vi "ep_Compute Third Current (SGL WFM).vi"(0 "current waveforms in":waveform(sgl)[](array[waveform]), 5 "wiring":T1, 11 "error in (no error)":errorcluster) -> (4 "current waveforms out":waveform(sgl)[](array[waveform]), 15 "error out":errorcluster)   [LabVIEW 2011, in "NI_EP_Power Quality.lvlib"]
uses:
  <vilib>/addons/Electrical Power/PQ/NI_EP_Power Quality.lvlib
  <vilib>/addons/Electrical Power/PQ/Common/Controls/ep_Wiring.ctl
  <vilib>/addons/Electrical Power/PQ/Common/Controls/ep_AI Data Channel.ctl
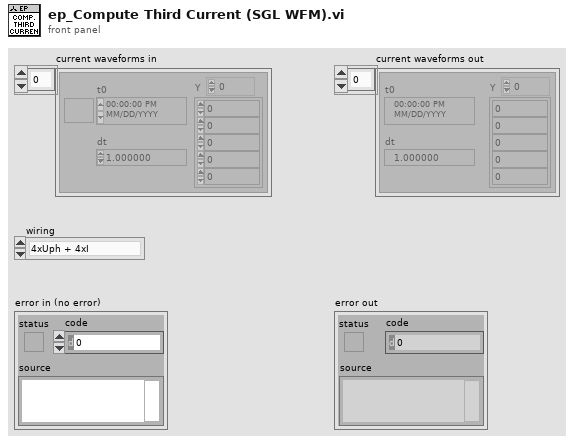
[diagram p1: front panel]
types:
  T1 = typedef "NI_EP_Power Quality.lvlib/ep_Wiring.ctl" = enum16{"4xUph + 4xI", "3xUph + 4xI", "3xUline + 4xI", "3xUph + 3xI", "3xUline + 3xI", "3xUph + 2xI", "3xUline + 2xI", "1xUph + 1xI"}
  T2 = typedef "NI_EP_Power Quality.lvlib/ep_AI Data Channel.ctl" = enum16{"Voltage Phase A (L1)", "Voltage Phase B (L2)", "Voltage Phase C (L3)", "Voltage Phase N (Neutral)", "Current Phase A (L1)", "Current Phase B (L2)", "Current Phase C (L3)", "Current Phase N (Neutral)"}
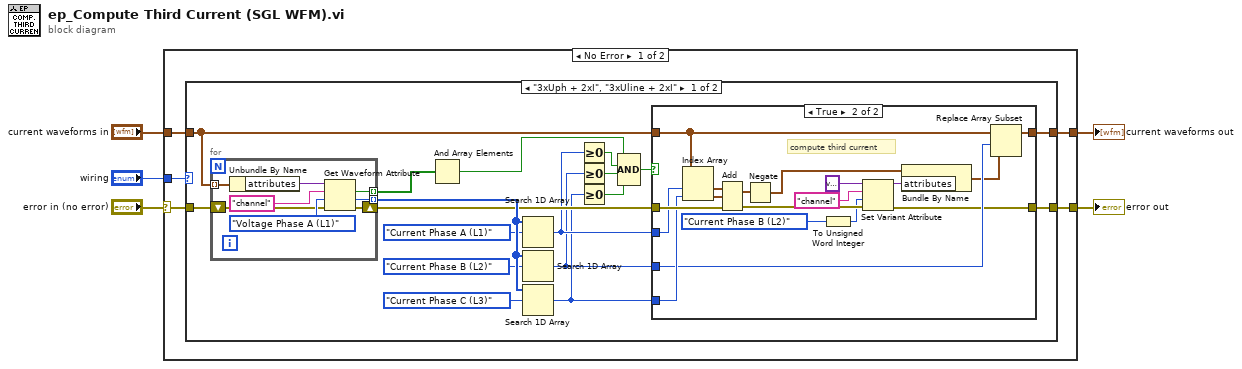
[diagram p0: block diagram]
diagram:
  n1 = case shown="No Error" "error in (no error)" {
    selector: "error in (no error)" -> [w6 w59]
    tunnel: "wiring" -> [w10 _]
    tunnel: [w9 w59] -> w4
    tunnel: [w8 _] -> w3
    tunnel: "current waveforms in" -> [w7 _]
    frame No Error {
      n2 = case shown="\"3xUph + 2xI\", \"3xUline + 2xI\"" w10 {
        tunnel: w7 -> [w13 w58]
        tunnel: [w28 w58] -> w8
        tunnel: w6 -> [w18 w57]
        tunnel: [w27 w57] -> w9
        frame "3xUph + 2xI", "3xUline + 2xI" {
          n3 = for {
            tunnel: w13 -> [w56] mode=indexing
            tunnel: [w52] -> w23 mode=indexing
            shift-right: [w50] -> w19
            shift-left: w18 -> [w51]
            tunnel: [w49] -> w12 mode=indexing
            n4 = Unbundle By Name(w56) -> ("attributes"=w55:variant)
            n5 = Get Waveform Attribute(4:w51, 5:ep_AI_Data_Channel."Voltage Phase A (L1)" ("AI data channel"), 6:"channel" ("name"), 7:w55) -> (0:w50:errorcluster, 1:w52:T2, 2:w49:bool)  [unwired: 1 out]
          }
          n6 = And Array Elements(Boolean array=w12) -> (logical AND=w11:bool)
          n7 = Search 1D Array(1D array=w23, element=ep_AI_Data_Channel."Current Phase A (L1)" ("AI data channel")) -> (index of element=w16:i32)  [unwired: 1 in]
          n8 = Search 1D Array(1D array=w23, element=ep_AI_Data_Channel."Current Phase B (L2)" ("AI data channel")) -> (index of element=w14:i32)  [unwired: 1 in]
          n9 = Search 1D Array(1D array=w23, element=ep_AI_Data_Channel."Current Phase C (L3)" ("AI data channel")) -> (index of element=w15:i32)  [unwired: 1 in]
          n10 = Greater Or Equal To 0?(x=w16) -> (x >= 0?=w24:bool)
          n11 = Greater Or Equal To 0?(x=w14) -> (x >= 0?=w25:bool)
          n12 = Greater Or Equal To 0?(x=w15) -> (x >= 0?=w26:bool)
          n13 = Compound Arithmetic op=AND(w11, w24, w25, w26) -> (w17:bool)
          n14 = case shown="True" w17 {
            tunnel: [w29 w45] -> w28
            tunnel: [w30 w35] -> w27
            tunnel: w13 -> [w29 w44]
            tunnel: w19 -> [w30 w43]
            tunnel: w16 -> [_ w42]
            tunnel: w15 -> [_ w41]
            tunnel: w14 -> [_ w40]
            frame False {
            }
            frame True {
              # "compute third current"
              n15 = Index Array(array=w44, index #1=w42, index #2=w41) -> (element #1=w48:waveform(sgl), element #2=w47:waveform(sgl))
              n16 = Add(1:w47, 2:w48, 4:w43) -> (0:w46:waveform(sgl), 3:w36:errorcluster)
              n17 = Negate(x=w46) -> (-x=w39:waveform(sgl))
              n18 = To Unsigned Word Integer(number=ep_AI_Data_Channel."Current Phase B (L2)" ("AI data channel")) -> (unsigned 16bit integer=w31:u16)
              n19 = Set Variant Attribute(Variant=variant ("variant"), name="channel", value=w31, error in=w36) -> (Variant out=w34:variant, error out=w35:errorcluster)  [unwired: 1 out]
              n20 = Bundle By Name(cluster=w39, "attributes"=w34) -> (w33:waveform(sgl))
              n21 = Replace Array Subset(array=w44, new element=w33, index=w40) -> (w45:waveform(sgl)[])
            }
          }
        }
        frame Default {
        }
      }
    }
    frame Error {
    }
  }
  "error out" <- w4
  "current waveforms out" <- w3
